vi "S2DS_DetermineTargetNew.vi"(3 "Scan parameters  in":T1 {"Y data taking" items=["in both direction", "in up direction only", "in down direction only"]; "X data taking" items=["in both direction", "in up direction only", "in down direction only"]}) -> (0 "Change  x direction":bool, 1 "Scan parameters  out":T1 {"Y data taking" items=["in both direction", "in up direction only", "in down direction only"]; "X data taking" items=["in both direction", "in up direction only", "in down direction only"]})   [LabVIEW 2016]
uses:
  TYPE DEFS/S2DS_Sweep Info.ctl
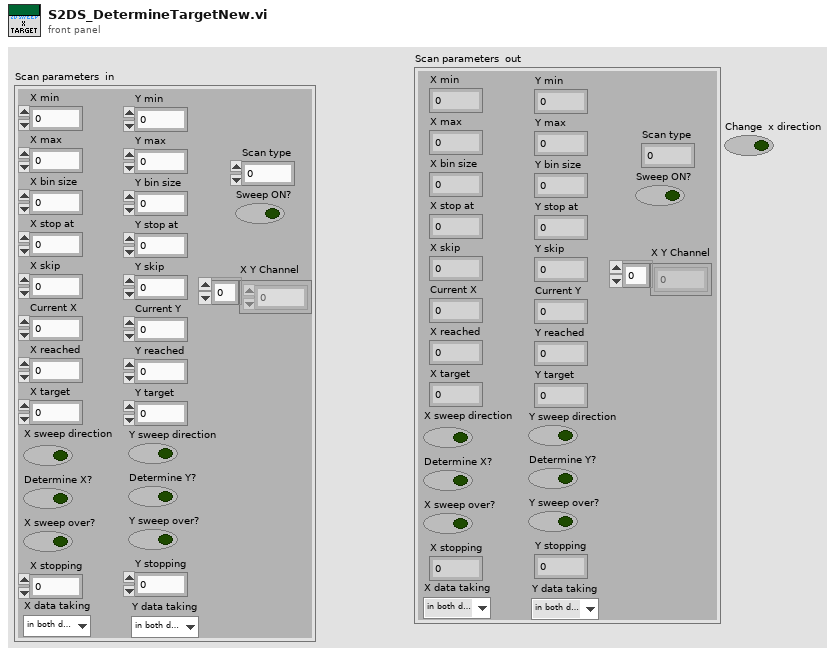
[diagram p1: front panel]
types:
  T1 = typedef "S2DS_Sweep Info.ctl" = cluster{"X min":ext, "X max":dbl, "Y min":dbl, "Y max":dbl, "X bin size":dbl, "Y bin size":dbl, "X stop at":dbl, "Y stop at":dbl, "X skip":u64, "Y skip":u64, "Current X":dbl, "Current Y":dbl, "X reached":i32, "Y reached":i32, "X target":dbl, "Y target":dbl, "Sweep ON?":bool, "X sweep direction":bool, "Y sweep direction":bool, "Determine X?":bool, "Determine Y?":bool, "X sweep over?":bool, "Y sweep over?":bool, "Scan type":i32, "X stopping":i32, "Y stopping":i32, "X Y Channel":u16[], "X data taking":u16, "Y data taking":u16}
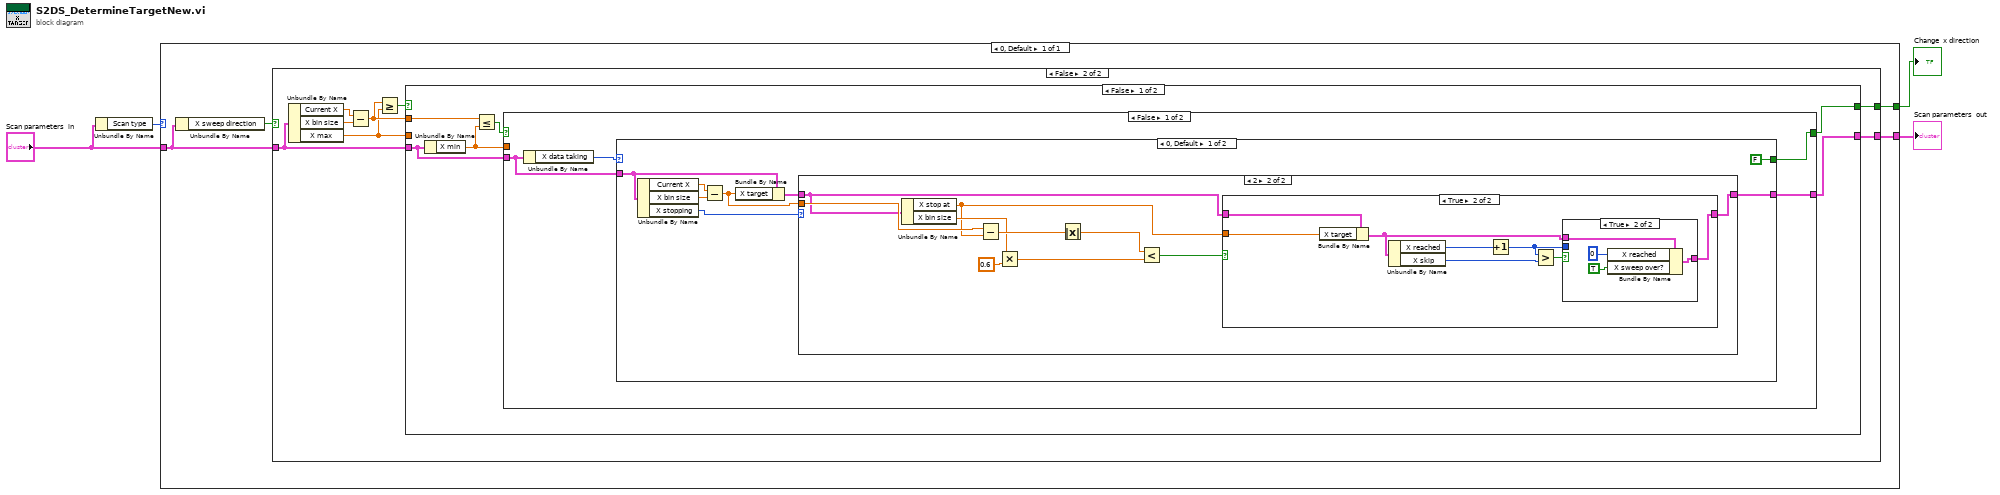
[diagram p0: block diagram]
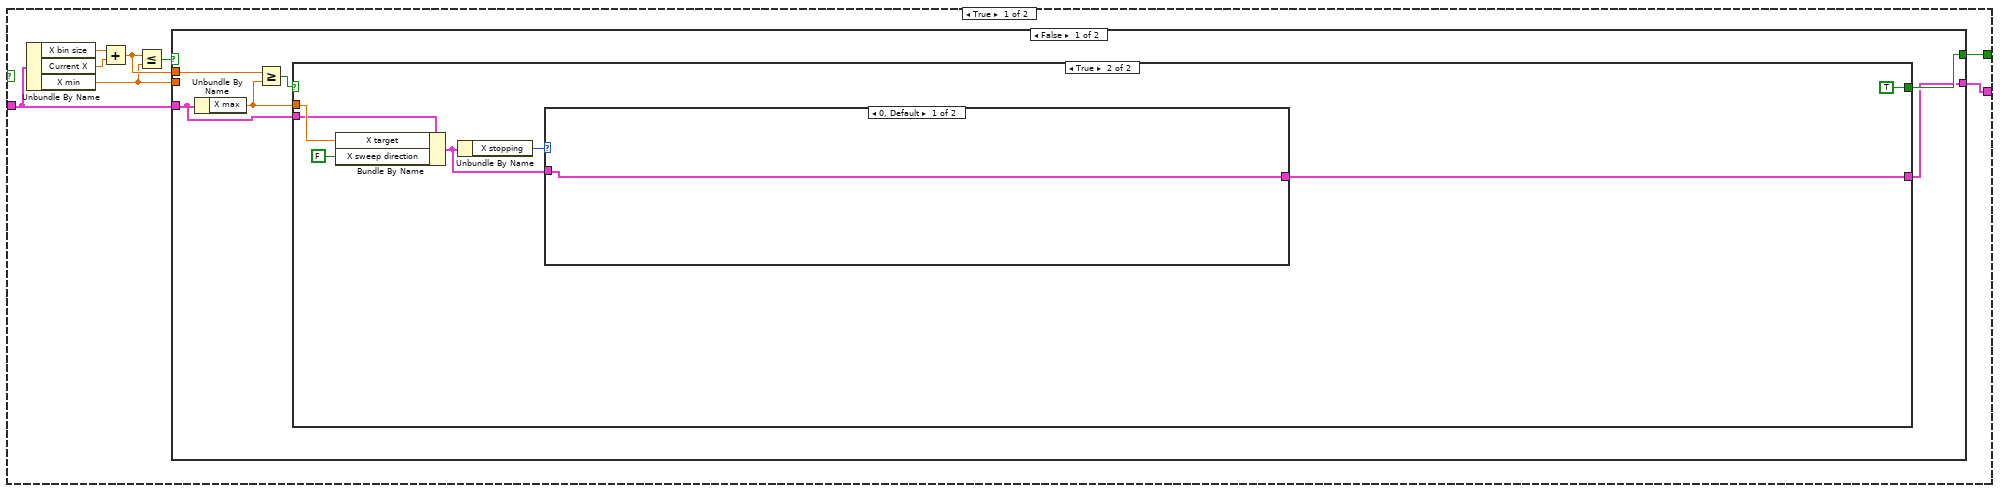
[diagram p2: hidden frame]
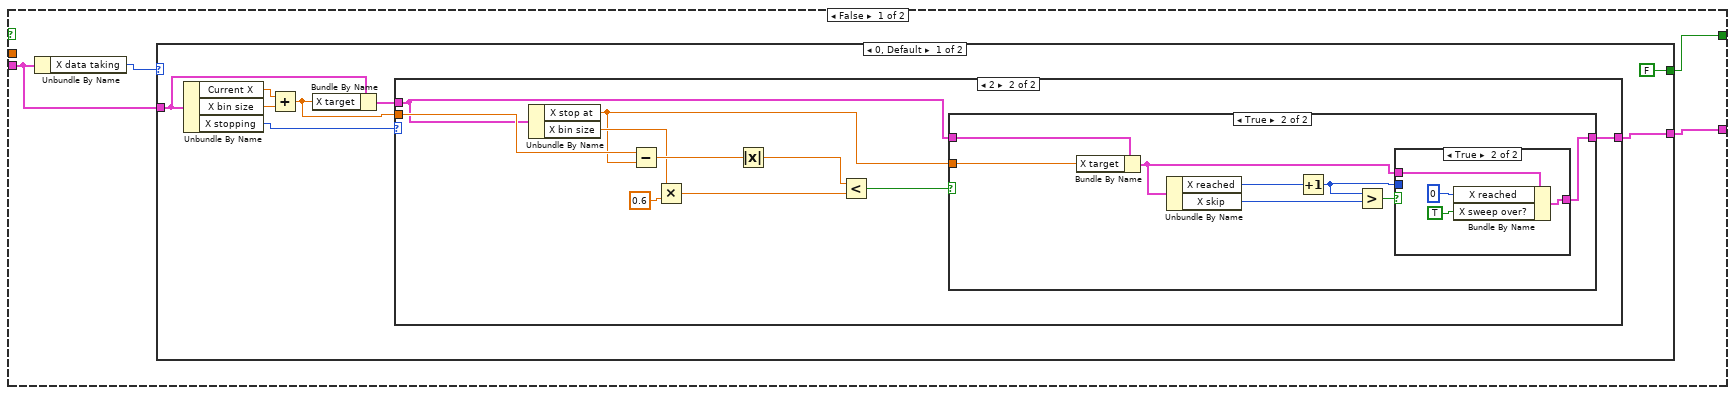
[diagram p3: hidden frame]
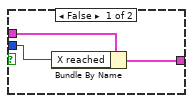
[diagram p6: hidden frame]
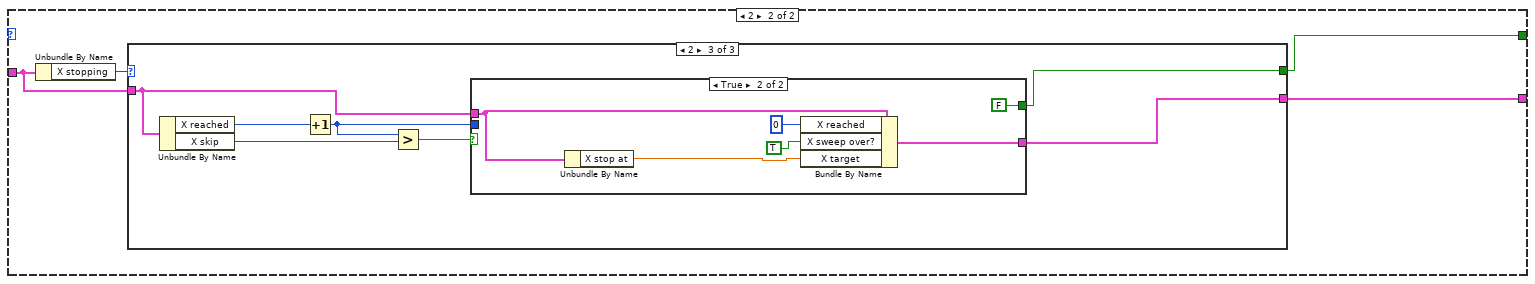
[diagram p7: hidden frame]
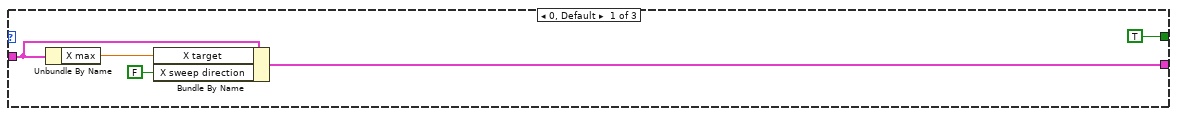
[diagram p8: hidden frame]
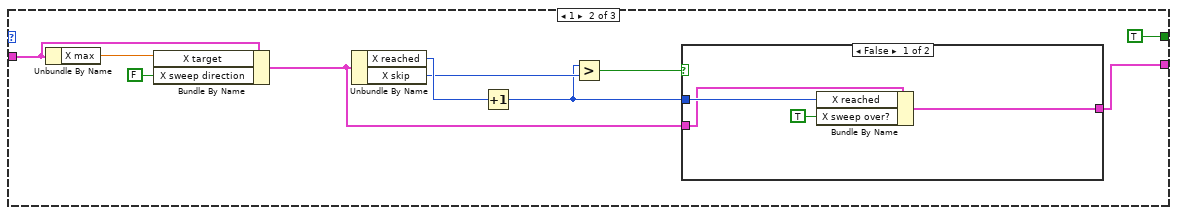
[diagram p9: hidden frame]
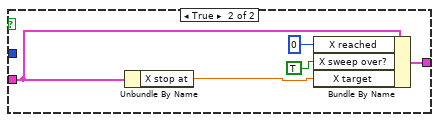
[diagram p10: hidden frame]
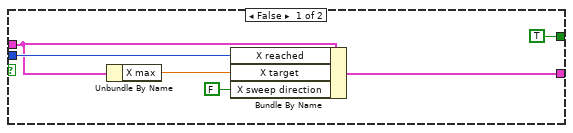
[diagram p11: hidden frame]
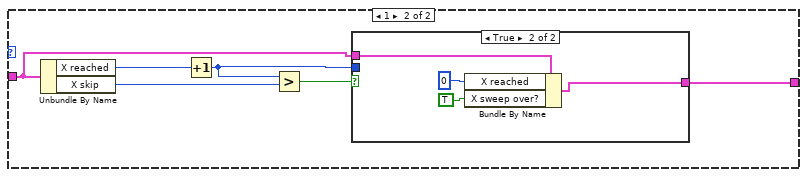
[diagram p12: hidden frame]
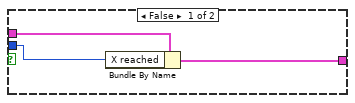
[diagram p13: hidden frame]
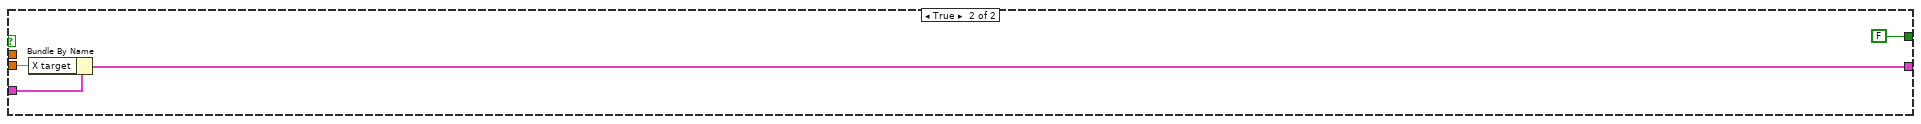
[diagram p14: hidden frame]
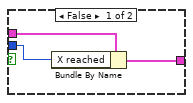
[diagram p17: hidden frame]
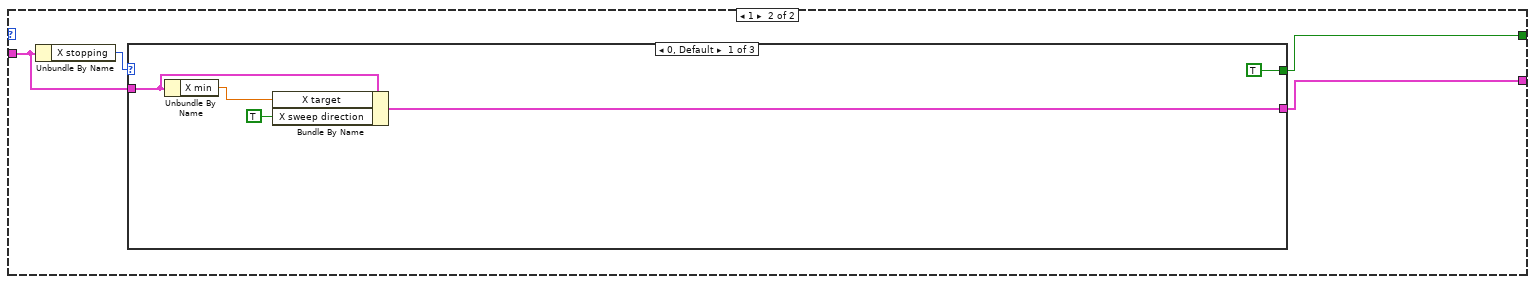
[diagram p18: hidden frame]
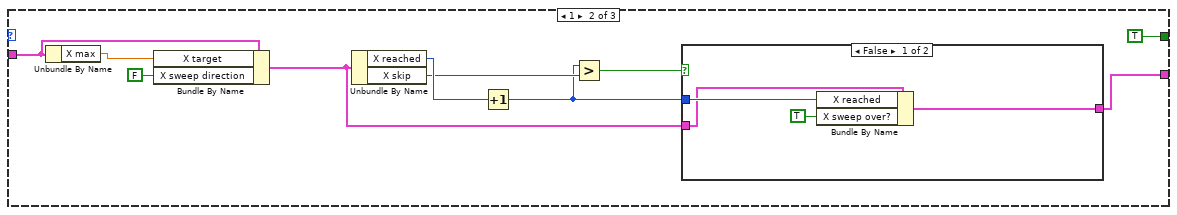
[diagram p19: hidden frame]
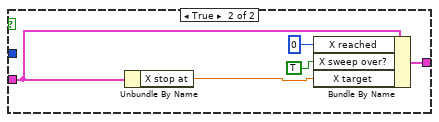
[diagram p20: hidden frame]
diagram:
  n1 = Unbundle By Name("Scan parameters  in") -> ("Scan type"=w4:i32)
  n2 = case shown="0, Default" w4 {
    tunnel: "Scan parameters  in" -> [w8]
    tunnel: [w6] -> w2
    tunnel: [w5] -> w1
    frame 0, Default {
      n3 = Unbundle By Name(w8) -> ("X sweep direction"=w7:bool)
      n4 = case shown="False" w7 {
        tunnel: w8 -> [w14 w139]
        tunnel: [w10 w135] -> w6
        tunnel: [w9 w134] -> w5
        frame True {
          n5 = Unbundle By Name(w14) -> ("X bin size"=w16:dbl, "Current X"=w15:dbl, "X min"=w11:ext)
          n6 = Add(x=w16, y=w15) -> (x+y=w12:dbl)
          n7 = Less Or Equal?(x=w12, y=w11) -> (x <= y?=w13:bool)
          n8 = case shown="False" w13 {
            tunnel: w14 -> [w20 w133]
            tunnel: w12 -> [w22 _]
            tunnel: [w17 w132] -> w9
            tunnel: w11 -> [_ w131]
            tunnel: [w18 FALSE] -> w10
            frame False {
              n9 = Unbundle By Name(w20) -> ("X max"=w19:dbl)
              n10 = Greater Or Equal?(x=w22, y=w19) -> (x >= y?=w21:bool)
              n11 = case shown="True" w21 {
                tunnel: w20 -> [w25 w113]
                tunnel: w19 -> [_ w115]
                tunnel: [w23 TRUE] -> w18
                tunnel: [w24 w109] -> w17
                frame False {
                  n12 = Unbundle By Name(w25) -> ("X data taking"=w26:u16)
                  n13 = case shown="0, Default" w26 {
                    tunnel: w25 -> [w32 w64]
                    tunnel: [w28 w62] -> w24
                    tunnel: [FALSE w63] -> w23
                    frame 0, Default {
                      n14 = Unbundle By Name(w32) -> ("Current X"=w34:dbl, "X bin size"=w33:dbl, "X stopping"=w31:i32)
                      n15 = Add(x=w34, y=w33) -> (x+y=w29:dbl)
                      n16 = Bundle By Name(cluster=w32, "X target"=w29) -> (w30:T1)
                      n17 = case shown="2" w31 {
                        tunnel: w30 -> [w35 w39]
                        tunnel: w29 -> [_ w45]
                        tunnel: [w35 w36] -> w28
                        frame 0, Default {
                        }
                        frame 2 {
                          n18 = Unbundle By Name(w39) -> ("X stop at"=w38:dbl, "X bin size"=w42:dbl)
                          n19 = Subtract(x=w45, y=w38) -> (x-y=w44:dbl)
                          n20 = Multiply(x=w42, y=0.6) -> (x*y=w40:dbl)
                          n21 = Absolute Value(x=w44) -> (abs(x)=w43:dbl)
                          n22 = Less?(x=w43, y=w40) -> (x < y?=w37:bool)
                          n23 = case shown="True" w37 {
                            tunnel: w39 -> [w46 w49]
                            tunnel: w38 -> [_ w54]
                            tunnel: [w46 w47] -> w36
                            frame False {
                            }
                            frame True {
                              n24 = Bundle By Name(cluster=w49, "X target"=w54) -> (w48:T1)
                              n25 = Unbundle By Name(w48) -> ("X reached"=w53:i32, "X skip"=w52:u64)
                              n26 = Increment(x=w53) -> (x+1=w50:i32)
                              n27 = Greater?(x=w50, y=w52) -> (0:w51:bool)
                              n28 = case shown="True" w51 {
                                tunnel: w50 -> [w56 _]
                                tunnel: w48 -> [w57 w61]
                                tunnel: [w55 w58] -> w47
                                frame False {
                                n29 = Bundle By Name(cluster=w57, "X reached"=w56) -> (w55:T1)
                                }
                                frame True {
                                n30 = Bundle By Name(cluster=w61, "X reached"=0, "X sweep over?"=TRUE) -> (w58:T1)
                                }
                              }
                            }
                          }
                        }
                      }
                    }
                    frame 2 {
                      n31 = Unbundle By Name(w64) -> ("X stopping"=w65:i32)
                      n32 = case shown="2" w65 {
                        tunnel: w64 -> [w70 w80 w92]
                        tunnel: [w66 w71 w91] -> w62
                        tunnel: [TRUE TRUE w90] -> w63
                        frame 0, Default {
                          n33 = Unbundle By Name(w70) -> ("X max"=w68:dbl)
                          n34 = Bundle By Name(cluster=w70, "X target"=w68, "X sweep direction"=FALSE) -> (w66:T1)
                        }
                        frame 1 {
                          n35 = Unbundle By Name(w80) -> ("X max"=w78:dbl)
                          n36 = Bundle By Name(cluster=w80, "X target"=w78, "X sweep direction"=FALSE) -> (w72:T1)
                          n37 = Unbundle By Name(w72) -> ("X reached"=w76:i32, "X skip"=w75:u64)
                          n38 = Increment(x=w76) -> (x+1=w73:i32)
                          n39 = Greater?(x=w73, y=w75) -> (0:w74:bool)
                          n40 = case shown="False" w74 {
                            tunnel: w73 -> [w84 _]
                            tunnel: w72 -> [w82 w86]
                            tunnel: [w83 w87] -> w71
                            frame False {
                              n41 = Bundle By Name(cluster=w82, "X reached"=w84, "X sweep over?"=TRUE) -> (w83:T1)
                            }
                            frame True {
                              n42 = Unbundle By Name(w86) -> ("X stop at"=w85:dbl)
                              n43 = Bundle By Name(cluster=w86, "X reached"=0, "X sweep over?"=TRUE, "X target"=w85) -> (w87:T1)
                            }
                          }
                        }
                        frame 2 {
                          n44 = Unbundle By Name(w92) -> ("X reached"=w96:i32, "X skip"=w95:u64)
                          n45 = Increment(x=w96) -> (x+1=w93:i32)
                          n46 = Greater?(x=w93, y=w95) -> (0:w94:bool)
                          n47 = case shown="True" w94 {
                            tunnel: w93 -> [w102 _]
                            tunnel: w92 -> [w100 w105]
                            tunnel: [w101 w106] -> w91
                            tunnel: [TRUE FALSE] -> w90
                            frame False {
                              n48 = Unbundle By Name(w100) -> ("X max"=w99:dbl)
                              n49 = Bundle By Name(cluster=w100, "X reached"=w102, "X target"=w99, "X sweep direction"=FALSE) -> (w101:T1)
                            }
                            frame True {
                              n50 = Unbundle By Name(w105) -> ("X stop at"=w104:dbl)
                              n51 = Bundle By Name(cluster=w105, "X reached"=0, "X sweep over?"=TRUE, "X target"=w104) -> (w106:T1)
                            }
                          }
                        }
                      }
                    }
                  }
                }
                frame True {
                  n52 = Bundle By Name(cluster=w113, "X target"=w115, "X sweep direction"=FALSE) -> (w111:T1)
                  n53 = Unbundle By Name(w111) -> ("X stopping"=w112:i32)
                  n54 = case shown="0, Default" w112 {
                    tunnel: w111 -> [w116 w118]
                    tunnel: [w116 w117] -> w109
                    frame 0, Default {
                    }
                    frame 1 {
                      n55 = Unbundle By Name(w118) -> ("X reached"=w122:i32, "X skip"=w121:u64)
                      n56 = Increment(x=w122) -> (x+1=w119:i32)
                      n57 = Greater?(x=w119, y=w121) -> (0:w120:bool)
                      n58 = case shown="True" w120 {
                        tunnel: w119 -> [w124 _]
                        tunnel: w118 -> [w125 w129]
                        tunnel: [w123 w126] -> w117
                        frame False {
                          n59 = Bundle By Name(cluster=w125, "X reached"=w124) -> (w123:T1)
                        }
                        frame True {
                          n60 = Bundle By Name(cluster=w129, "X reached"=0, "X sweep over?"=TRUE) -> (w126:T1)
                        }
                      }
                    }
                  }
                }
              }
            }
            frame True {
              n61 = Bundle By Name(cluster=w133, "X target"=w131) -> (w132:T1)
            }
          }
        }
        frame False {
          n62 = Unbundle By Name(w139) -> ("Current X"=w141:dbl, "X bin size"=w140:dbl, "X max"=w136:dbl)
          n63 = Subtract(x=w141, y=w140) -> (x-y=w137:dbl)
          n64 = Greater Or Equal?(x=w137, y=w136) -> (x >= y?=w138:bool)
          n65 = case shown="False" w138 {
            tunnel: w139 -> [w145 w258]
            tunnel: w137 -> [w147 _]
            tunnel: [w142 w257] -> w134
            tunnel: w136 -> [_ w256]
            tunnel: [w143 FALSE] -> w135
            frame False {
              n66 = Unbundle By Name(w145) -> ("X min"=w144:ext)
              n67 = Less Or Equal?(x=w147, y=w144) -> (x <= y?=w146:bool)
              n68 = case shown="False" w146 {
                tunnel: w145 -> [w150 w238]
                tunnel: w144 -> [_ w240]
                tunnel: [w148 TRUE] -> w143
                tunnel: [w149 w234] -> w142
                frame False {
                  n69 = Unbundle By Name(w150) -> ("X data taking"=w151:u16)
                  n70 = case shown="0, Default" w151 {
                    tunnel: w150 -> [w157 w189]
                    tunnel: [w153 w187] -> w149
                    tunnel: [FALSE w188] -> w148
                    frame 0, Default {
                      n71 = Unbundle By Name(w157) -> ("Current X"=w159:dbl, "X bin size"=w158:dbl, "X stopping"=w156:i32)
                      n72 = Subtract(x=w159, y=w158) -> (x-y=w154:dbl)
                      n73 = Bundle By Name(cluster=w157, "X target"=w154) -> (w155:T1)
                      n74 = case shown="2" w156 {
                        tunnel: w155 -> [w160 w164]
                        tunnel: w154 -> [_ w170]
                        tunnel: [w160 w161] -> w153
                        frame 0, Default {
                        }
                        frame 2 {
                          n75 = Unbundle By Name(w164) -> ("X stop at"=w163:dbl, "X bin size"=w167:dbl)
                          n76 = Subtract(x=w170, y=w163) -> (x-y=w169:dbl)
                          n77 = Multiply(x=w167, y=0.6) -> (x*y=w165:dbl)
                          n78 = Absolute Value(x=w169) -> (abs(x)=w168:dbl)
                          n79 = Less?(x=w168, y=w165) -> (x < y?=w162:bool)
                          n80 = case shown="True" w162 {
                            tunnel: w164 -> [w171 w174]
                            tunnel: w163 -> [_ w179]
                            tunnel: [w171 w172] -> w161
                            frame False {
                            }
                            frame True {
                              n81 = Bundle By Name(cluster=w174, "X target"=w179) -> (w173:T1)
                              n82 = Unbundle By Name(w173) -> ("X reached"=w178:i32, "X skip"=w177:u64)
                              n83 = Increment(x=w178) -> (x+1=w175:i32)
                              n84 = Greater?(x=w175, y=w177) -> (0:w176:bool)
                              n85 = case shown="True" w176 {
                                tunnel: w175 -> [w181 _]
                                tunnel: w173 -> [w182 w186]
                                tunnel: [w180 w183] -> w172
                                frame False {
                                n86 = Bundle By Name(cluster=w182, "X reached"=w181) -> (w180:T1)
                                }
                                frame True {
                                n87 = Bundle By Name(cluster=w186, "X reached"=0, "X sweep over?"=TRUE) -> (w183:T1)
                                }
                              }
                            }
                          }
                        }
                      }
                    }
                    frame 1 {
                      n88 = Unbundle By Name(w189) -> ("X stopping"=w190:i32)
                      n89 = case shown="0, Default" w190 {
                        tunnel: w189 -> [w195 w205 w217]
                        tunnel: [w191 w196 w216] -> w187
                        tunnel: [TRUE TRUE w215] -> w188
                        frame 0, Default {
                          n90 = Unbundle By Name(w195) -> ("X min"=w193:ext)
                          n91 = Bundle By Name(cluster=w195, "X target"=w193, "X sweep direction"=TRUE) -> (w191:T1)
                        }
                        frame 1 {
                          n92 = Unbundle By Name(w205) -> ("X max"=w203:dbl)
                          n93 = Bundle By Name(cluster=w205, "X target"=w203, "X sweep direction"=FALSE) -> (w197:T1)
                          n94 = Unbundle By Name(w197) -> ("X reached"=w201:i32, "X skip"=w200:u64)
                          n95 = Increment(x=w201) -> (x+1=w198:i32)
                          n96 = Greater?(x=w198, y=w200) -> (0:w199:bool)
                          n97 = case shown="False" w199 {
                            tunnel: w198 -> [w209 _]
                            tunnel: w197 -> [w207 w211]
                            tunnel: [w208 w212] -> w196
                            frame False {
                              n98 = Bundle By Name(cluster=w207, "X reached"=w209, "X sweep over?"=TRUE) -> (w208:T1)
                            }
                            frame True {
                              n99 = Unbundle By Name(w211) -> ("X stop at"=w210:dbl)
                              n100 = Bundle By Name(cluster=w211, "X reached"=0, "X sweep over?"=TRUE, "X target"=w210) -> (w212:T1)
                            }
                          }
                        }
                        frame 2 {
                          n101 = Unbundle By Name(w217) -> ("X reached"=w221:i32, "X skip"=w220:u64)
                          n102 = Increment(x=w221) -> (x+1=w218:i32)
                          n103 = Greater?(x=w218, y=w220) -> (0:w219:bool)
                          n104 = case shown="False" w219 {
                            tunnel: w218 -> [w227 _]
                            tunnel: w217 -> [w225 w230]
                            tunnel: [w226 w231] -> w216
                            tunnel: [TRUE FALSE] -> w215
                            frame False {
                              n105 = Unbundle By Name(w225) -> ("X min"=w224:ext)
                              n106 = Bundle By Name(cluster=w225, "X reached"=w227, "X target"=w224, "X sweep direction"=TRUE) -> (w226:T1)
                            }
                            frame True {
                              n107 = Unbundle By Name(w230) -> ("X stop at"=w229:dbl)
                              n108 = Bundle By Name(cluster=w230, "X reached"=0, "X sweep over?"=TRUE, "X target"=w229) -> (w231:T1)
                            }
                          }
                        }
                      }
                    }
                  }
                }
                frame True {
                  n109 = Bundle By Name(cluster=w238, "X target"=w240, "X sweep direction"=TRUE) -> (w236:T1)
                  n110 = Unbundle By Name(w236) -> ("X stopping"=w237:i32)
                  n111 = case shown="0, Default" w237 {
                    tunnel: w236 -> [w241 w243]
                    tunnel: [w241 w242] -> w234
                    frame 0, Default {
                    }
                    frame 1 {
                      n112 = Unbundle By Name(w243) -> ("X reached"=w247:i32, "X skip"=w246:u64)
                      n113 = Increment(x=w247) -> (x+1=w244:i32)
                      n114 = Greater?(x=w244, y=w246) -> (0:w245:bool)
                      n115 = case shown="False" w245 {
                        tunnel: w244 -> [w249 _]
                        tunnel: w243 -> [w250 w254]
                        tunnel: [w248 w251] -> w242
                        frame False {
                          n116 = Bundle By Name(cluster=w250, "X reached"=w249) -> (w248:T1)
                        }
                        frame True {
                          n117 = Bundle By Name(cluster=w254, "X reached"=0, "X sweep over?"=TRUE) -> (w251:T1)
                        }
                      }
                    }
                  }
                }
              }
            }
            frame True {
              n118 = Bundle By Name(cluster=w258, "X target"=w256) -> (w257:T1)
            }
          }
        }
      }
    }
  }
  "Scan parameters  out" <- w1
  "Change  x direction" <- w2
